vi "rad_Configure Target Dialog.vi"(5 "Password":string, 8 "Error In":errorcluster, 11 "Target Information in":T1={"Hostname"="", "Serial number"="", "Product name"="", "Product code"=0, "System status"="", "Credential type"=enum."None/Unlocked", "User added?"=FALSE, "Primary NIC"={"MAC address"="", "IP Address Request Mode"=2, "IP address"="", "Subnet mask"="", "Gateway"="", "DNS server"=""}} {"Primary NIC"."IP Address Request Mode" items=["Static"=1, "DHCP/Link-Local"=2, "Link-Local Only"=4, "DHCP Only"=8]}) -> (0 "Error Out":errorcluster, 3 "Target Information out":T1={"Hostname"="", "Serial number"="", "Product name"="", "Product code"=0, "System status"="", "Credential type"=enum."None/Unlocked", "User added?"=FALSE, "Primary NIC"={"MAC address"="", "IP Address Request Mode"=2, "IP address"="", "Subnet mask"="", "Gateway"="", "DNS server"=""}} {"Primary NIC"."IP Address Request Mode" items=["Static"=1, "DHCP/Link-Local"=2, "Link-Local Only"=4, "DHCP Only"=8]})   [LabVIEW 2020]
uses:
  TypeDefs/rad_Target Information.ctl
  TypeDefs/rad_Target Network Settings.ctl
panel:
  in  "IP Address Request Mode":i32(ring)=2 items=["Static"=1, "DHCP/Link-Local"=2, "Link-Local Only"=4, "DHCP Only"=8]
  in  "DNS":string
  in  "Gateway":string
  in  "Subnet Mask":string
  in  "IP Address":string
  in  "Host Name":string
  in  "Cancel":bool
  in  "OK":bool
  # "Network Configuration"
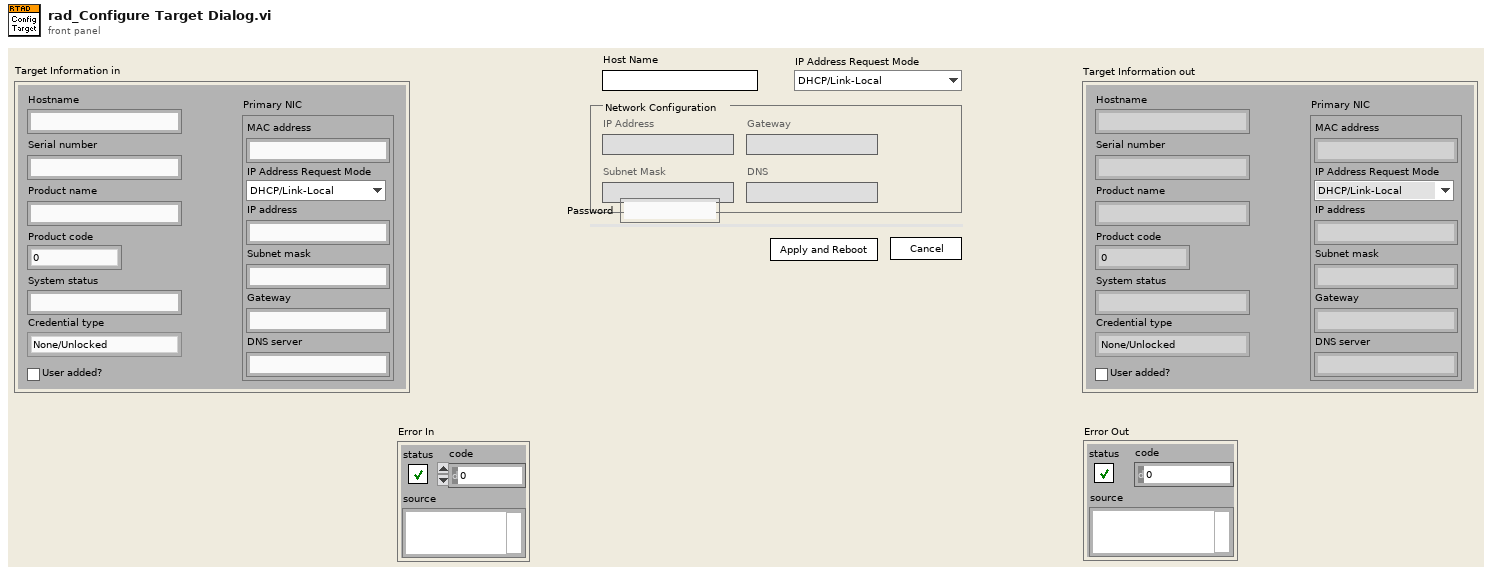
[diagram p1: front panel]
types:
  T1 = typedef "rad_Target Information.ctl" = cluster{"Hostname":string, "Serial number":string, "Product name":string, "Product code":i32, "System status":string, "Credential type":enum16{"None/Unlocked", "FTP Password", "NIAuth Credentials"}, "User added?":bool, "Primary NIC":T2}
  T2 = typedef "rad_Target Network Settings.ctl" = cluster{"MAC address":string, "IP Address Request Mode":i32, "IP address":string, "Subnet mask":string, "Gateway":string, "DNS server":string}
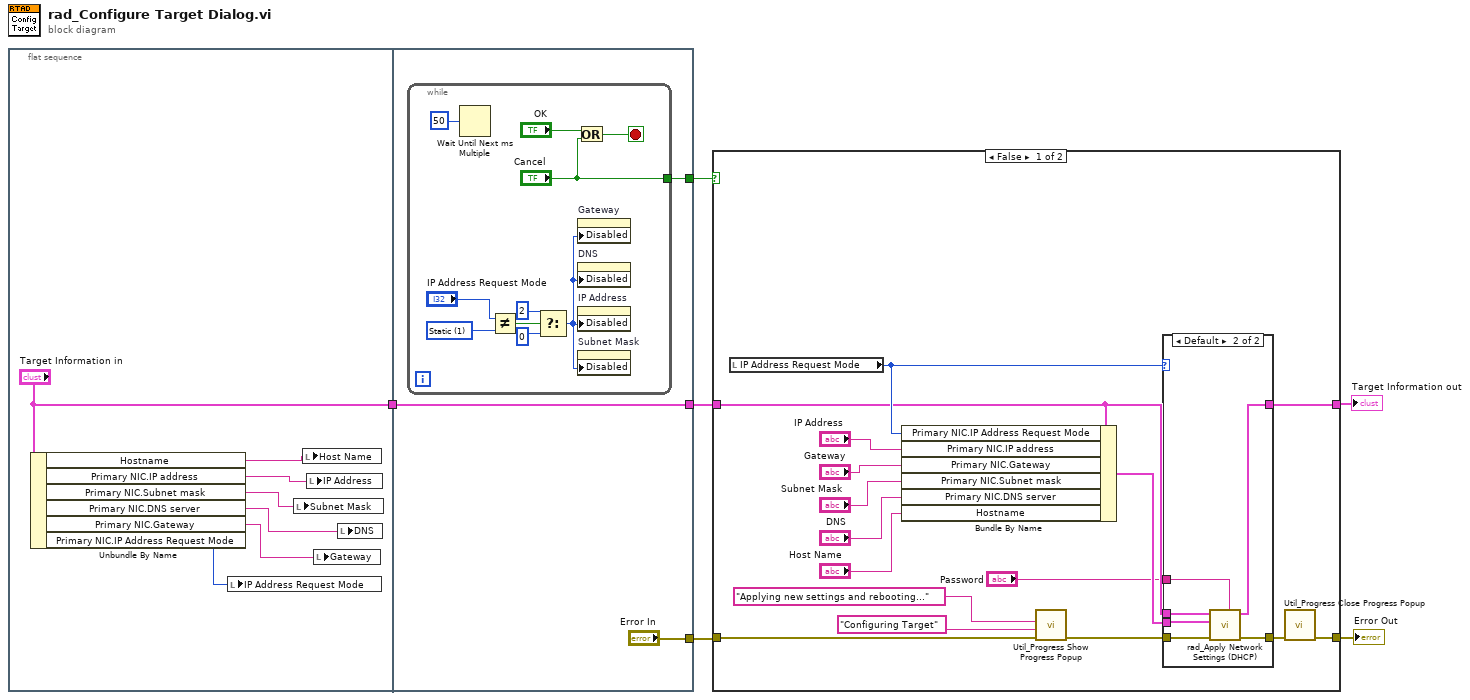
[diagram p0: block diagram]
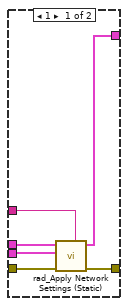
[diagram p2: hidden frame]
diagram:
  n1 = flat-sequence {
    tunnel: ["Target Information in"] -> w6
    tunnel: w6 -> [w15]
    tunnel: [w16] -> w3
    tunnel: [w15] -> w2
    tunnel: ["Error In"] -> w1
    frame #0 {
      n2 = Unbundle By Name("Target Information in") -> ("Hostname"=w13:string, "Primary NIC.IP address"=w12:string, "Primary NIC.Subnet mask"=w11:string, "Primary NIC.DNS server"=w10:string, "Primary NIC.Gateway"=w9:string, "Primary NIC.IP Address Request Mode"=w7:i32)
      n3 = local write "IP Address Request Mode"(w7) -> ()
      n4 = local write "Subnet Mask"(w11) -> ()
      n5 = local write "Host Name"(w13) -> ()
      n6 = local write "IP Address"(w12) -> ()
      n7 = local write "Gateway"(w9) -> ()
      n8 = local write "DNS"(w10) -> ()
    }
    frame #1 {
      n9 = while {
        tunnel: ["Cancel"] -> w16
        stop <- w24 stop-if-true
        w18 = 1 items=["Static"=1, "DHCP/Link-Local"=2, "Link-Local Only"=4, "DHCP Only"=8] ("IP Address Request Mode")
        n10 = Wait Until Next ms Multiple(millisecond multiple=u32 50) -> ()  [unwired: 1 out]
        n11 = Not Equal?(x="IP Address Request Mode", y=w18) -> (x != y?=w17:bool)
        n12 = Select(t=u8 2 ("Disabled"), s=w17, f=u8 0 ("Disabled")) -> (s? t:f=w20:u8)
        n13 = Or(x="OK", y="Cancel") -> (x .or. y?=w24:bool)
        n14 = property on="Gateway" class="Str"("Disabled"=w20) -> ()  [unwired: 2 in, 2 out]
        n15 = property on="DNS" class="Str"("Disabled"=w20) -> ()  [unwired: 2 in, 2 out]
        n16 = property on="IP Address" class="Str"("Disabled"=w20) -> ()  [unwired: 2 in, 2 out]
        n17 = property on="Subnet Mask" class="Str"("Disabled"=w20) -> ()  [unwired: 2 in, 2 out]
      }
    }
  }
  n18 = case shown="False" w3 {
    tunnel: w2 -> [w28 w56]
    tunnel: [w29 w56] -> w4
    tunnel: [w37 w55] -> w5
    tunnel: w1 -> [w40 w55]
    frame False {
      n19 = local read "IP Address Request Mode"() -> (w32:i32)
      n20 = Bundle By Name(cluster=w28, "Primary NIC.IP Address Request Mode"=w32, "Primary NIC.IP address"="IP Address", "Primary NIC.Gateway"="Gateway", "Primary NIC.Subnet mask"="Subnet Mask", "Primary NIC.DNS server"="DNS", "Hostname"="Host Name") -> (w31:T1)
      n21 = call "Util_Progress Show Progress Popup.vi"("error in (no error)"=w40, "Title"="Configuring Target", "Message"="Applying new settings and rebooting...") -> ("error out"=w38:errorcluster)  [unwired: 1 in, 7 out]
      n22 = case shown="Default" w32 {
        tunnel: [w47 w53] -> w39
        tunnel: w38 -> [w48 w54]
        tunnel: w31 -> [w45 w51]
        tunnel: [w44 w52] -> w29
        tunnel: w28 -> [w46 w50]
        tunnel: "Password" -> [w43 w49]
        frame 1 {
          n23 = call "rad_Apply Network Settings (Static).vi"("Password"=w43, "error in (no error)"=w48, "Requested settings"=w45, "Existing settings"=w46) -> ("error out"=w47:errorcluster, "Target settings out"=w44:T1)  [unwired: 6 in]
        }
        frame Default {
          n24 = call "rad_Apply Network Settings (DHCP).vi"("Password"=w49, "error in (no error)"=w54, "Requested settings"=w51, "Existing settings"=w50) -> ("error out"=w53:errorcluster, "Target settings out"=w52:T1)  [unwired: 6 in]
        }
      }
      n25 = call "Util_Progress Close Progress Popup.vi"("error in (no error)"=w39) -> ("error out"=w37:errorcluster)  [unwired: 2 in, 8 out]
    }
    frame True {
    }
  }
  "Target Information out" <- w4
  "Error Out" <- w5
